vi "Insert Control into Map.vi"(9 "Ctl Data":T1, 10 "Name":string, 11 "Control Map":map{string, T1[]}(c390)) -> (3 "Control Map out":map{string, T1[]}(c390))   [LabVIEW 2020, in "MacroAssert.lvlib"]
doc: "Inserts the control identified by <B>Name</B> into <B>Control Map</B> along with its related <B>Ctl Data</B>."
uses:
  MacroAssert.lvlib
  CTLs/Control Map Control Data.ctl
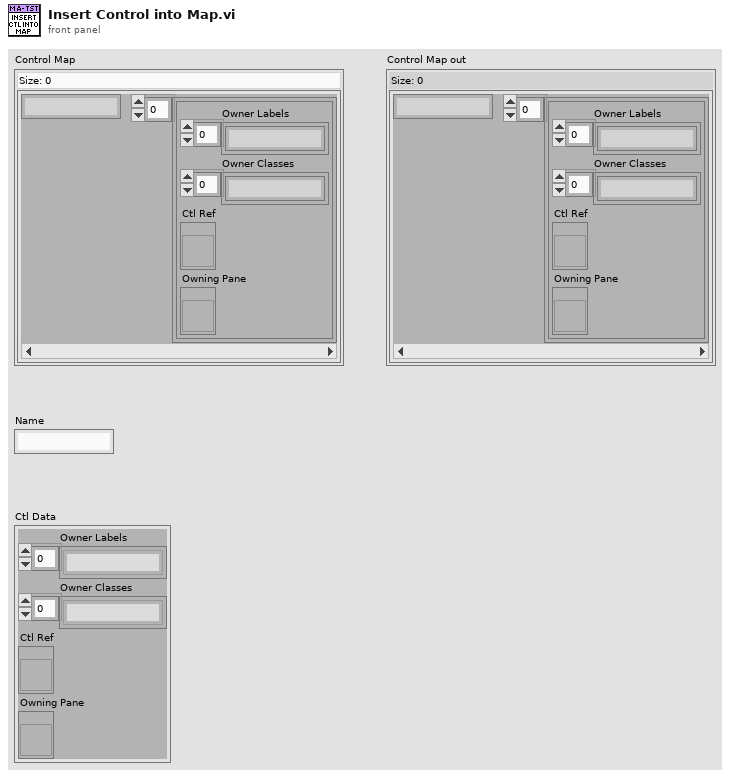
[diagram p1: front panel]
types:
  T1 = typedef "MacroAssert.lvlib/Control Map Control Data.ctl" = cluster{"Owner Labels":string[], "Owner Classes":string[], "Ctl Ref":refnum<vi>, "Owning Pane":refnum<vi>}
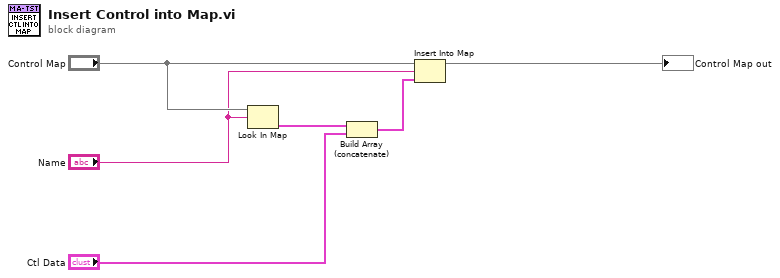
[diagram p0: block diagram]
diagram:
  n1 = Look In Map(map="Control Map", key="Name") -> (value=w4:T1[])  [unwired: 1 in, 1 out]
  n2 = Build Array (concatenate)(w4, "Ctl Data") -> (w2:T1[])
  n3 = Insert Into Map(map in="Control Map", key="Name", value=w2) -> (map out=→"Control Map out":map{string, T1[]})  [unwired: 2 out]
